vi "AB_Engine_Compute_Toplevel_Implied_Links.vi"(10 "File":T2, 11 "Linker:Read Info From File":T3(array[cluster])) -> (0 "All owned instance VIs can exclude front panel?":bool, 1 "links":u32[](array[numeric]))   [LabVIEW 2020]
doc: "This VI adds all owned instance VI and private data control links to our links (recursively), and checks to see if ourselves or any VI whose links we are assuming require us to keep our front panel"
uses:
  <vilib>/Utility/lvfile.llb/LVFileType.ctl
  <vilib>/AppBuilder/AB_Classes/Source/AB_Source.lvclass
  <vilib>/Utility/lvfile.llb/NI_FileType.lvlib
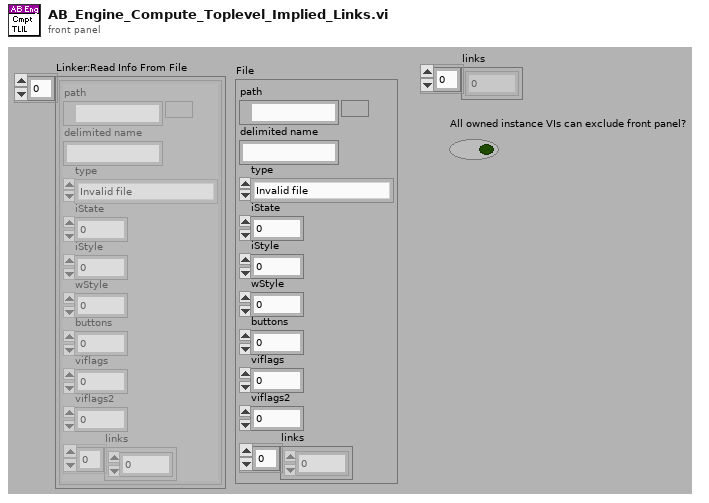
[diagram p1: front panel]
types:
  T1 = typedef "NI_FileType.lvlib/LVFileType.ctl" = enum32{"Invalid file", "Unknown type", "Instrument", "Control", "Polymorphic VI", "Project", "Library", "LVClass", "XControl", "XNode", "Shared library", ".NET assembly", "ActiveX interface", "CIN", "Run-time menu", "Palette menu", "Help file", "LLB", "XNode Edit Dependency", "Class Private Data Control", "Statechart", "MathScript .m file", "Ladder Diagram", "LVLibp", "XNode Build Dependency"}
  T2 = cluster{"path":path, "delimited name":string, "type":T1, "iState":u32, "iStyle":u16, "wStyle":u16, "buttons":u16, "viflags":u32, "viflags2":u32, "links":u32[]}
  T3 = cluster{"path":path, "delimited name":string, "type":T1, "iState":u32, "iStyle":u16, "wStyle":u16, "buttons":u16, "viflags":u32, "viflags2":u32, "links":u32[]}[]
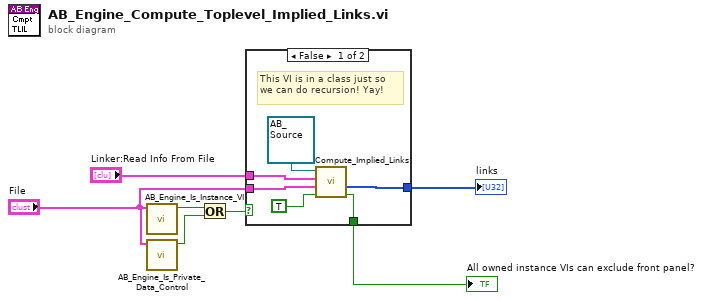
[diagram p0: block diagram]
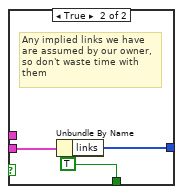
[diagram p2: hidden frame]
diagram:
  n1 = call <vilib>:"AB_Engine_Is_Instance_VI.vi"("File"="File") -> ("Is Instance VI?"=w7:bool)  [unwired: 10 in]
  n2 = call <vilib>:"AB_Engine_Is_Private_Data_Control.vi"("File"="File") -> ("Is Private Data Control?"=w6:bool)  [unwired: 10 in]
  n3 = Or(x=w7, y=w6) -> (x .or. y?=w5:bool)
  n4 = case shown="False" w5 {
    tunnel: "File" -> [w11 w16]
    tunnel: "Linker:Read Info From File" -> [w10 _]
    tunnel: [w9 w14] -> w2
    tunnel: [w8 TRUE ("Exclude front panel? (false if not checking)")] -> w1
    frame False {
      # "This VI is in a class just so we can do recursion! Yay!"
      n5 = call-dynamic "Compute_Implied_Links.vi"("Check front panel exclusion?"=TRUE, "File"=w11, "Linker:Read Info From File"=w10, "AB_Source.lvclass"=refnum<class "AB_Source.lvclass"> refnum) -> ("Exclude front panel? (false if not checking)"=w8:bool, "links"=w9:u32[])  [unwired: 6 in]
    }
    frame True {
      # "Any implied links we have are assumed by our owner, so don't waste time with them"
      n6 = Unbundle By Name(w16) -> ("links"=w14:u32[])
    }
  }
  "links" <- w2
  "All owned instance VIs can exclude front panel?" <- w1
